vi "Channel Settings to CDO.vi"(10 "channel settings":T4[](array[typedef]), 11 "drive from slot":T1) -> (1 "channel default values":dbl[](array[numeric]), 2 "channel names":string[](array[string]), 3 "CDO":T2)   [LabVIEW 2017, in "Scan Engine Scripting.lvlib"]
uses:
  Scan Engine Scripting.lvlib
  Modules/Mode Classes/Controls/counter driven output channel settings.ctl
  Modules/Channel Classes/Counter Driven Output Channel/Counter Driven State.ctl
  Modules.lvlibp/SD Module/Type Defs/CDO.ctl
  Modules.lvlibp/SD Module/Type Defs/CDO Channel.ctl
  Modules/Mode Classes/Counter Driven Output Mode/Drive from Slot.ctl
  Modules.lvlibp/SD Module/SD Module.lvclass
  Modules/Channel Classes/Counter Driven Output Channel/Counter Driven Output Channel.lvclass
  Modules/Mode Classes/Counter Driven Output Mode/Counter Driven Output Mode.lvclass
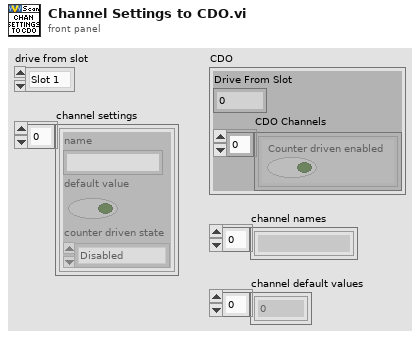
[diagram p1: front panel]
types:
  T1 = typedef "Scan Engine Scripting.lvlib/Counter Driven Output Mode.lvclass/Drive from Slot.ctl" = enum16{"Slot 1", "Slot 2", "Slot 3", "Slot 4", "Slot 5", "Slot 6", "Slot 7", "Slot 8"}
  T2 = typedef "Modules.lvlibp/SD Module.lvclass/CDO.ctl" = cluster{"Drive From Slot":u32, "CDO Channels":T3[]}
  T3 = typedef "Modules.lvlibp/SD Module.lvclass/CDO Channel.ctl" = cluster{"Counter driven enabled":bool}
  T4 = typedef "Scan Engine Scripting.lvlib/counter driven output channel settings.ctl" = cluster{"name":string, "default value":bool, "counter driven state":T5}
  T5 = typedef "Scan Engine Scripting.lvlib/Counter Driven Output Channel.lvclass/Counter Driven State.ctl" = enum16{"Disabled", "Enabled"}
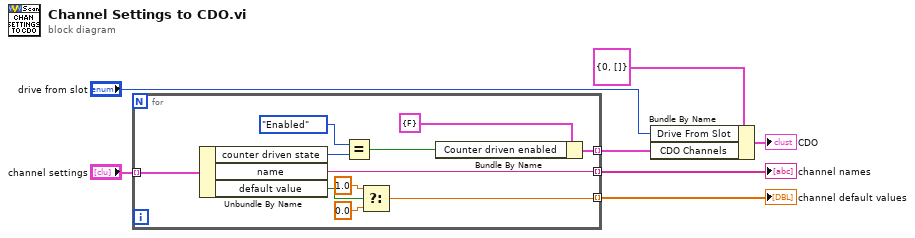
[diagram p0: block diagram]
diagram:
  n1 = for {
    tunnel: "channel settings" -> [w18] mode=indexing
    tunnel: [w13] -> w4 mode=indexing
    tunnel: [w12] -> w6 mode=indexing
    tunnel: [w8] -> w7 mode=indexing
    n2 = Unbundle By Name(w18) -> ("counter driven state"=w16:T5, "name"=w12:string, "default value"=w10:bool)
    n3 = Equal?(x=Counter_Driven_State."Enabled", y=w16) -> (x = y?=w14:bool)
    n4 = Select(t=1.0, s=w10, f=0.0) -> (s? t:f=w8:dbl)
    n5 = Bundle By Name(cluster=T3 {"Counter driven enabled"=FALSE} ("CDO Channel"), "Counter driven enabled"=w14) -> (w13:T3)
  }
  "channel default values" <- w7
  "channel names" <- w6
  n6 = Bundle By Name(cluster=T2 {"Drive From Slot"=0, "CDO Channels"=[]} ("CDO"), "Drive From Slot"="drive from slot", "CDO Channels"=w4) -> (→"CDO":T2)
